vi "Get Instance.vi"(5 "error in (no error)":errorcluster caption="错误输入（无错误）") -> (14 "reference out":refnum<class "Single.lvclass">, 19 "error out":errorcluster caption="错误输出")   [LabVIEW 2013, in "Single.lvclass"]
uses:
  Single.lvclass
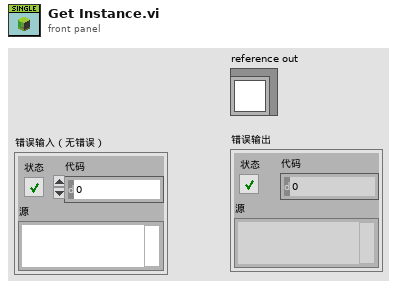
[diagram p1: front panel]
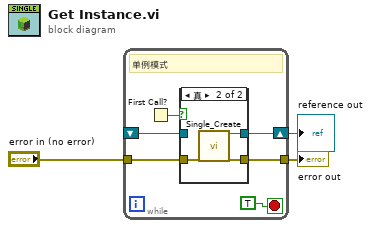
[diagram p0: block diagram]
diagram:
  n1 = while {
    shift-right: [w7] -> w1
    shift-left: _ -> [w6]
    tunnel: "error in (no error)" -> [w5]
    tunnel: [w4] -> w2
    stop <- TRUE stop-if-true
    # "单例模式"
    n2 = First Call?() -> (First Call?: T/F=w8:bool)
    n3 = case shown="真" w8 {
      tunnel: [w11 w14] -> w7
      tunnel: w6 -> [w11 _]
      tunnel: w5 -> [w10 w13]
      tunnel: [w10 w12] -> w4
      frame False {
      }
      frame True {
        n4 = call "Single_Create.vi"("error in (no error)"=w13) -> ("reference out"=w14:refnum<class "Single.lvclass">, "error out"=w12:errorcluster)  [unwired: 17 in]
      }
    }
  }
  "error out" <- w2
  "reference out" <- w1
